vi "64x48_Frame3.vi"   [LabVIEW 2014]
uses:
  QwaveSys_Interface/QwaveSys_Interface.lvlib
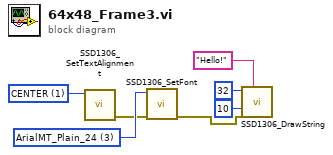
[diagram p0: block diagram]
diagram:
  w4 = u16 3 items=["Crushed_Plain_36", "ArialMT_Plain_10", "ArialMT_Plain_16", "ArialMT_Plain_24"] ("Font")
  w7 = u16 1 items=["LEFT", "CENTER", "RIGHT"] ("alignment")
  n1 = call "SSD1306_SetTextAlignment.vi"("alignment"=w7) -> ("error out"=w1:errorcluster)  [unwired: 10 in]
  n2 = call "SSD1306_SetFont.vi"("error in (no error)"=w1, "Font"=w4) -> ("error out"=w3:errorcluster)  [unwired: 9 in]
  n3 = call "SSD1306_DrawString.vi"("String"="Hello!", "error in (no error)"=w3, "y"=u8 10, "x"=u8 32) -> ()  [unwired: 7 in, 1 out]
